vi "Hardware - Setup and Arm Counter Task.vi"(1 "error in":errorcluster, 2 "CI.CountEdges.Term":tag="/Dev3/10MHzRefClock", 3 "Analog Task in":refnum<k21>="Dev7/ai0") -> (0 "error out":errorcluster)   [LabVIEW 2010, in "Core SubVIs.lvlib"]
uses:
  Core SubVIs.lvlib
  Controls/TYPE - Count Time Method.ctl
  <vilib>/DAQmx/configure/timing.llb/DAQmx Timing (Sample Clock).vi
  F:/Program Files/National Instruments/LabVIEW 2010/resource/objmgr/daqmx.rc
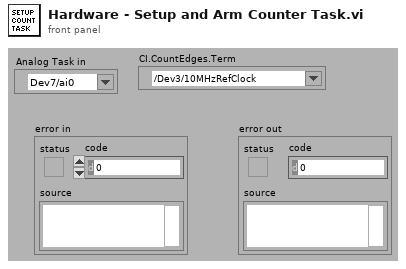
[diagram p1: front panel]
types:
  T1 = typedef "Core SubVIs.lvlib/TYPE - Count Time Method.ctl" = enum16{"Start Timer Task", "Read Timer", "Reset Timer", "Clear Timer Task"}
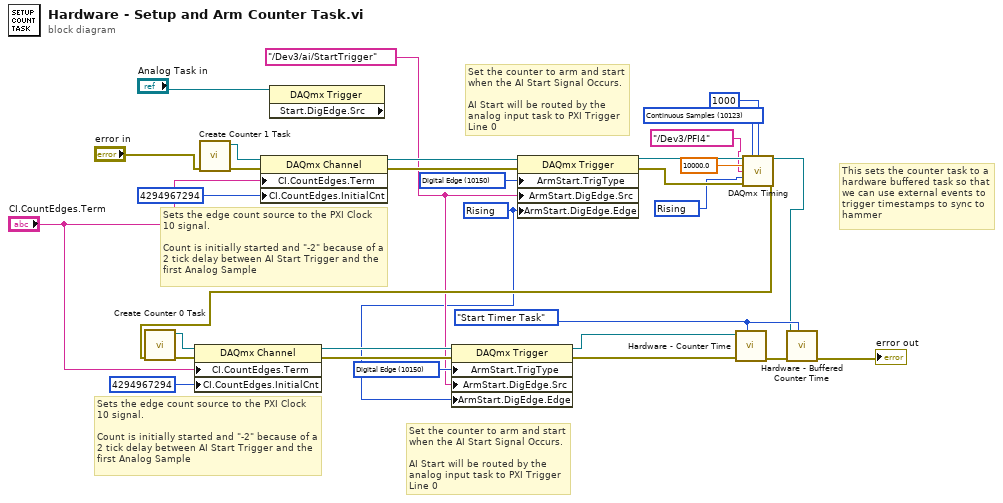
[diagram p0: block diagram]
diagram:
  w2 = 10280 items=["Rising"=10280, "Falling"=10171] ("active edge")
  w3 = 10280 items=["Rising"=10280, "Falling"=10171] ("ArmStart.DigEdge.Edge")
  w4 = tag "/Dev3/ai/StartTrigger" ("ArmStart.DigEdge.Src")
  w8 = 10150 items=["Digital Edge"=10150, "None"=10230] ("ArmStart.TrigType")
  w10 = 10123 items=["Finite Samples"=10178, "Continuous Samples"=10123, "Hardware Timed Single Point"=12522] ("sample mode")
  w16 = TYPE_-_Count_Time_Method."Start Timer Task" ("Counter Time Function (Read Timer)")
  w30 = 10150 items=["Digital Edge"=10150, "None"=10230] ("ArmStart.TrigType")
  # "Set the counter to arm and start when the AI Start Signal Occurs.\n\nAI Start will be routed by the analog input task to PXI Trigger Line 0"
  # "This sets the counter task to a \nhardware buffered task so that\nwe can use external events to\ntrigger timestamps to sync to\nhammer"
  # "Sets the edge count source to the PXI Clock 10 signal.\n\nCount is initially started and \"-2\" because of a 2 tick delay between AI Start Trigger and the first Analog Sample"
  # "Set the counter to arm and start when the AI Start Signal Occurs.\n\nAI Start will be routed by the analog input task to PXI Trigger Line 0"
  # "Sets the edge count source to the PXI Clock 10 signal.\n\nCount is initially started and \"-2\" because of a 2 tick delay between AI Start Trigger and the first Analog Sample"
  n1 = call "Create Counter 1 Task.vi"("error in"="error in") -> ("error out"=w22:errorcluster, "task out"=w21:refnum<k21>)  [unwired: 9 out]
  n2 = property class="DAQmx Channel"(reference=w21, error in=w22, "CI.CountEdges.Term"="CI.CountEdges.Term", "CI.CountEdges.InitialCnt"=u32 4294967294) -> (reference out=w23:refnum<k21>, error out=w24:errorcluster)
  n3 = property class="DAQmx Trigger" props=["Start.DigEdge.Src"](reference="Analog Task in") -> ()  [unwired: 1 in, 3 out]
  n4 = property class="DAQmx Trigger"(reference=w23, error in=w24, "ArmStart.TrigType"=w8, "ArmStart.DigEdge.Src"=w4, "ArmStart.DigEdge.Edge"=w3) -> (reference out=w14:refnum<k21>, error out=w15:errorcluster)
  n5 = call-poly <vilib>:"DAQmx Timing.vi"("task/channels in"=w14, "sample mode"=w10, "samples per channel"=1000, "rate"=10000.0, "source"=tag "/Dev3/PFI4", "active edge"=w2, "error in"=w15) -> ("task out"=w12:refnum<k21>, "error out"=w13:errorcluster)  [unwired: 7 out]
  n6 = call "Create Counter 0 Task.vi"("error in"=w13) -> ("error out"=w26:errorcluster, "task out"=w25:refnum<k21>)  [unwired: 9 out]
  n7 = property class="DAQmx Channel"(reference=w25, error in=w26, "CI.CountEdges.Term"="CI.CountEdges.Term", "CI.CountEdges.InitialCnt"=u32 4294967294) -> (reference out=w27:refnum<k21>, error out=w28:errorcluster)
  n8 = property class="DAQmx Trigger"(reference=w27, error in=w28, "ArmStart.TrigType"=w30, "ArmStart.DigEdge.Src"=w4, "ArmStart.DigEdge.Edge"=w3) -> (reference out=w31:refnum<k21>, error out=w6:errorcluster)
  n9 = call "Hardware - Counter Time.vi"("Counter Time Function (Read Timer)"=w16, "error in (no error)"=w6, "Counter Task In"=w31) -> ("error out"=w18:errorcluster)  [unwired: 8 out]
  n10 = call "Hardware - Buffered Counter Time.vi"("Counter Time Function (Read Timer)"=w16, "error in (no error)"=w18, "Counter Task In"=w12) -> ("error out"=→"error out":errorcluster)  [unwired: 8 out]
